vi "Formata_String.vi"(4 "entrada":string, 5 "Num de Caracteres":i32=2) -> (1 "saida":string)   [LabVIEW 2018]
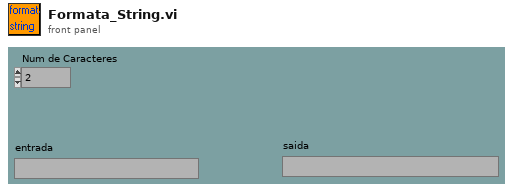
[diagram p1: front panel]
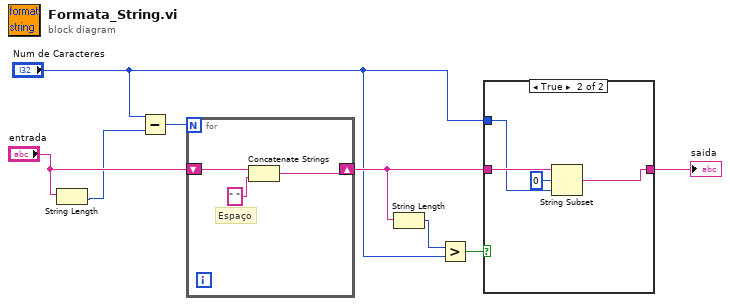
[diagram p0: block diagram]
diagram:
  n1 = String Length(string="entrada") -> (length=w7:i32)
  n2 = Subtract(x="Num de Caracteres", y=w7) -> (x-y=w6:i32)
  n3 = for {
    N: w6 -> [_]
    shift-right: [w10] -> w3
    shift-left: "entrada" -> [w11]
    # "Espaço"
    n4 = Concatenate Strings(w11, " " ("string")) -> (w10:string)
  }
  n5 = String Length(string=w3) -> (length=w5:i32)
  n6 = Greater?(x=w5, y="Num de Caracteres") -> (0:w4:bool)
  n7 = case shown="True" w4 {
    tunnel: [w12 w13] -> w1
    tunnel: w3 -> [w12 w16]
    tunnel: "Num de Caracteres" -> [_ w14]
    frame False {
    }
    frame True {
      n8 = String Subset(string=w16, offset (0)=0, length (rest)=w14) -> (substring=w13:string)
    }
  }
  "saida" <- w1
